vi "DisplacementCheckForTimeout.vi"(11 "DisplacementSampleSensorLoopData in":T1) -> (3 "DisplacementSampleSensorLoopData out":T1)   [LabVIEW 2018]
uses:
  DisplacementSampleSensorLoopData.ctl
  DisplacementSampleSensorLoopStates.ctl
  DisplacementSample.ctl
  DisplacementErrorSample.ctl
  DisplacementErrorCodes.ctl
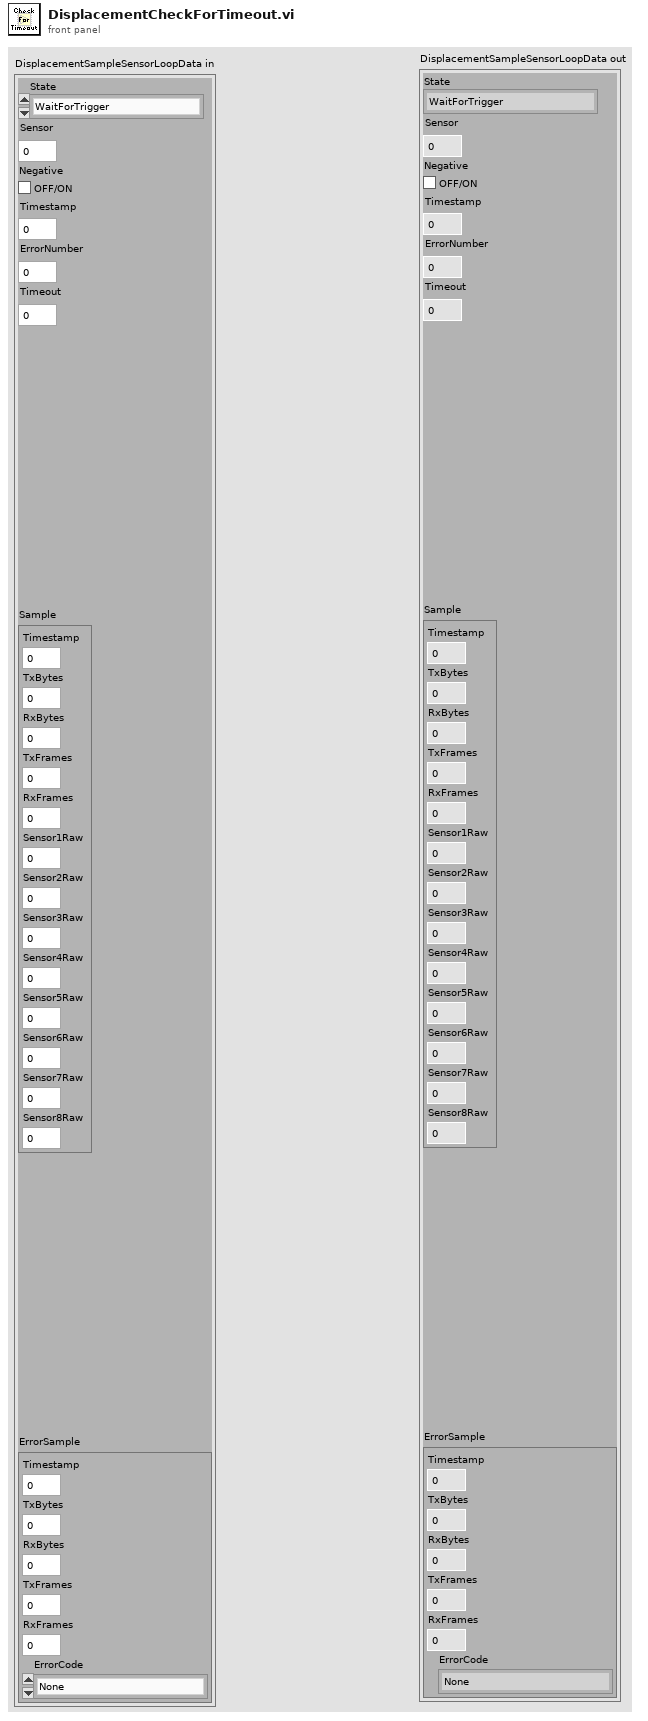
[diagram p1: front panel]
types:
  T1 = typedef "DisplacementSampleSensorLoopData.ctl" = cluster{"State":T2, "Sensor":u8, "Negative":bool, "Timestamp":u64, "ErrorNumber":u8, "Timeout":i32, "Sample":T3, "ErrorSample":T4}
  T2 = typedef "DisplacementSampleSensorLoopStates.ctl" = enum16{"WaitForTrigger", "ClearRxFIFO", "WaitForClearComplete", "WriteM", "Write0", "WriteCR", "WriteNL", "ReadFirstCharacter", "ReadDataResponse", "ReadDeliminator", "ReadSign", "ReadHundreds", "ReadTens", "ReadOnes", "ReadDecimal", "ReadTenths", "ReadHundredths", "ReadThousandths", "ReadTenThousandths", "ReadSampleNL", "PrepareSample", "MoveSample", "ReadErrorR", "ReadErrorDeliminator1", "ReadErrorM", "ReadError0", "ReadErrorDeliminator2", "ReadErrorNumberTens", "ReadErrorNumberOnes", "ReadErrorCR", "ReadErrorNL", "ParseErrorNumber", "ResponseUnknownError", "ResponseInvalidError", "ResponseTimeoutError", "SensorIndicatesInvalidCommandError", "SensorIndicatesCommunicationTimeoutError", "SensorIndicatesDataLengthError", "SensorIndicatesNumberOfParametersError", "SensorIndicatesParameterError", "SensorIndicatesCommunicationError", "SensorIndicatesIDNumberError", "SensorIndicatesExpansionLineError", "SensorIndicatesWriteControlError", "PrepareErrorCode", "MoveErrorCode"}
  T3 = typedef "DisplacementSample.ctl" = cluster{"Timestamp":u64, "TxBytes":u64, "RxBytes":u64, "TxFrames":u64, "RxFrames":u64, "Sensor1Raw":i32, "Sensor2Raw":i32, "Sensor3Raw":i32, "Sensor4Raw":i32, "Sensor5Raw":i32, "Sensor6Raw":i32, "Sensor7Raw":i32, "Sensor8Raw":i32}
  T4 = typedef "DisplacementErrorSample.ctl" = cluster{"Timestamp":u64, "TxBytes":u64, "RxBytes":u64, "TxFrames":u64, "RxFrames":u64, "ErrorCode":T5}
  T5 = typedef "DisplacementErrorCodes.ctl" = enum16{"None", "ResponseUnknownError", "ResponseInvalidError", "ResponseTimeoutError", "SensorIndicatesInvalidCommandError", "SensorIndicatesCommunicationTimeoutError", "SensorIndicatesDataLengthError", "SensorIndicatesNumberOfParametersError", "SensorIndicatesParameterError", "SensorIndicatesCommunicationError", "SensorIndicatesIDNumberError", "SensorIndicatesExpansionLineError", "SensorIndicatesWriteControlError"}
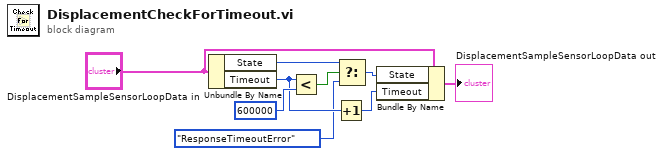
[diagram p0: block diagram]
diagram:
  n1 = Unbundle By Name("DisplacementSampleSensorLoopData in") -> ("State"=w1:T2, "Timeout"=w7:i32)
  n2 = Less?(x=w7, y=600000) -> (x < y?=w8:bool)
  n3 = Increment(x=w7) -> (x+1=w2:i32)
  n4 = Select(t=w1, s=w8, f=DisplacementSampleSensorLoopStates."ResponseTimeoutError") -> (s? t:f=w3:T2)
  n5 = Bundle By Name(cluster="DisplacementSampleSensorLoopData in", "State"=w3, "Timeout"=w2) -> (→"DisplacementSampleSensorLoopData out":T1)
